vi "popUPSeleccionReceta.vi"(9 "ingresarLote":string="numLote", 10 "ingresarSteelGrade":string="numSteelGrade", 11 "ingresarOD":string="numeroOD") -> (1 "idReceta":string, 2 "recetaSeleccionadaDeLaLista":string, 3 "Listo SeleccionListaDeReceta":bool=TRUE)   [LabVIEW 2014]
panel:
  in  "listaRecetas":i32(listbox)
  in  "textoFinCarga":string="Gracias por ingresar los datos del producto"
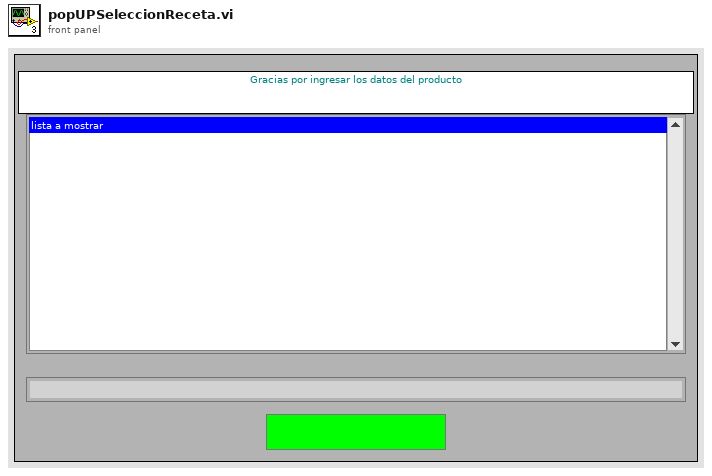
[diagram p1: front panel]
types:
  T1 = enum8{"Enabled", "Disabled", "Disabled and Grayed Out"}
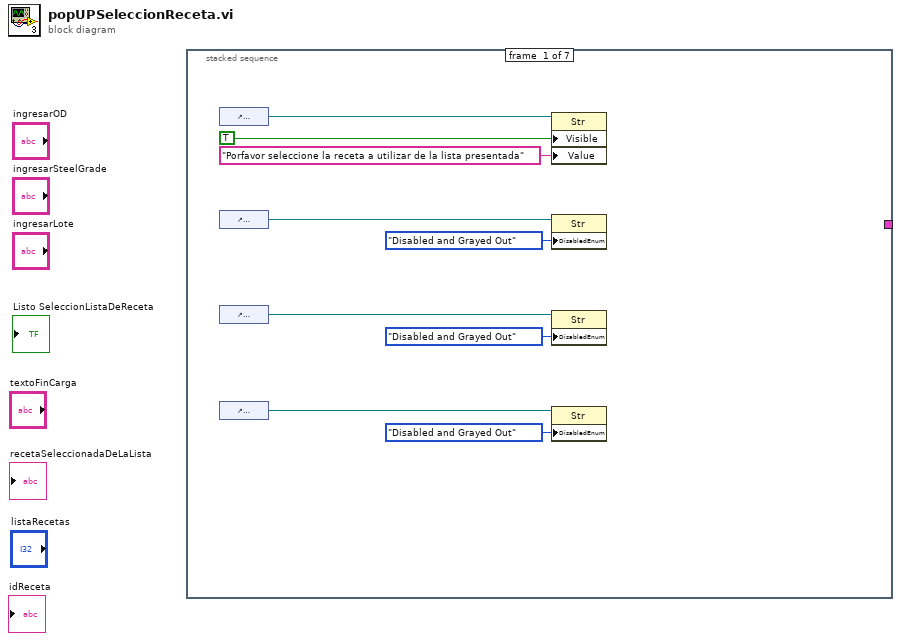
[diagram p0: block diagram]
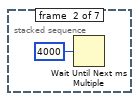
[diagram p2: hidden frame]
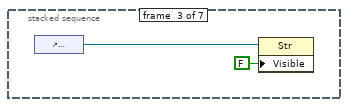
[diagram p3: hidden frame]
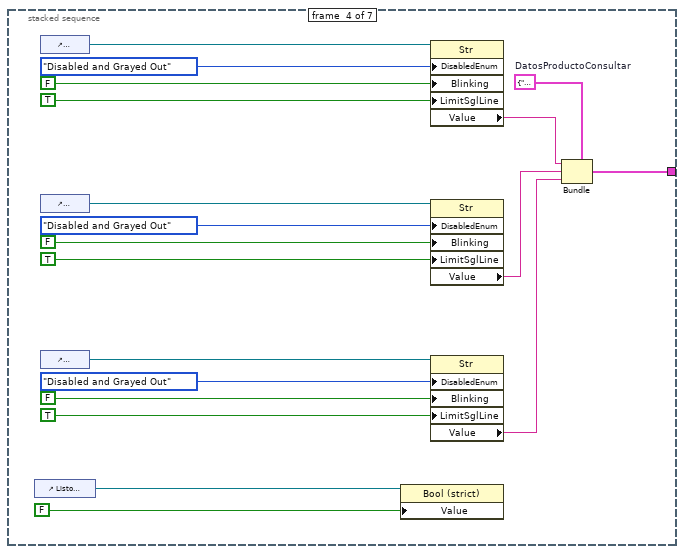
[diagram p4: hidden frame]
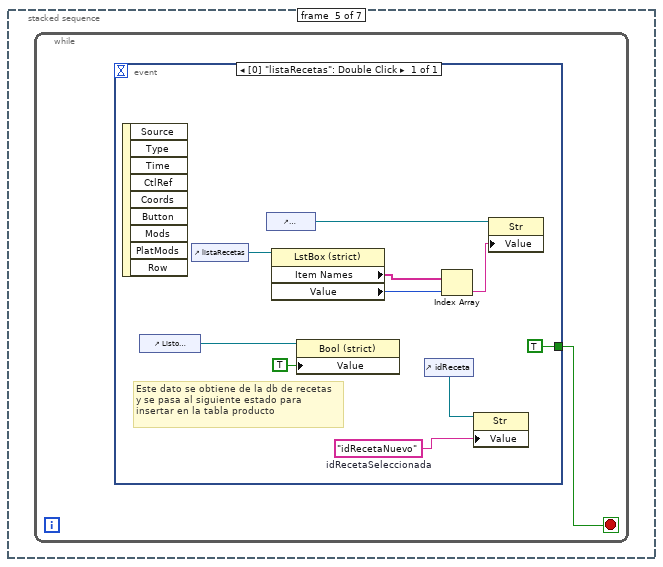
[diagram p5: hidden frame]
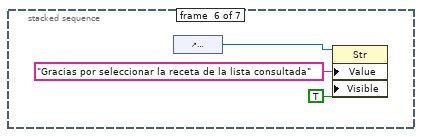
[diagram p6: hidden frame]
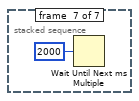
[diagram p7: hidden frame]
diagram:
  n1 = stacked-sequence {
    tunnel: [_ _ _ w13 _ _ _] -> _
    frame #0 {
      n2 = control-ref of="textoFinCarga"() -> (w9:refnum<vi>)
      n3 = control-ref of="ingresarOD"() -> (w6:refnum<vi>)
      n4 = control-ref of="ingresarSteelGrade"() -> (w5:refnum<vi>)
      n5 = control-ref of="ingresarLote"() -> (w4:refnum<vi>)
      n6 = property class="Str"(reference=w9, "Visible"=TRUE, "Value"="Porfavor seleccione la receta a utilizar de la lista presentada") -> ()  [unwired: 1 in, 2 out]
      n7 = property class="Str"(reference=w6, "DisabledEnum"=T1."Disabled and Grayed Out" ("Disabled")) -> ()  [unwired: 1 in, 2 out]
      n8 = property class="Str"(reference=w5, "DisabledEnum"=T1."Disabled and Grayed Out" ("Disabled")) -> ()  [unwired: 1 in, 2 out]
      n9 = property class="Str"(reference=w4, "DisabledEnum"=T1."Disabled and Grayed Out" ("Disabled")) -> ()  [unwired: 1 in, 2 out]
    }
    frame #1 {
      n10 = Wait Until Next ms Multiple(millisecond multiple=u32 4000) -> ()  [unwired: 1 out]
    }
    frame #2 {
      n11 = control-ref of="textoFinCarga"() -> (w12:refnum<vi>)
      n12 = property class="Str"(reference=w12, "Visible"=FALSE) -> ()  [unwired: 1 in, 2 out]
    }
    frame #3 {
      w14 = cluster{"OD":string, "SG":string, "LT":string} {"OD"="", "SG"="", "LT"=""}  # DatosProductoConsultar
      n13 = control-ref of="Listo SeleccionListaDeReceta"() -> (w19:refnum<vi>)
      n14 = control-ref of="ingresarOD"() -> (w31:refnum<vi>)
      n15 = control-ref of="ingresarSteelGrade"() -> (w29:refnum<vi>)
      n16 = control-ref of="ingresarLote"() -> (w27:refnum<vi>)
      n17 = property class="Bool (strict)"(reference=w19, "Value"=FALSE) -> ()  [unwired: 1 in, 2 out]
      n18 = property class="Str"(reference=w31, "DisabledEnum"=T1."Disabled and Grayed Out" ("Disabled"), "Blinking"=FALSE, "LimitSglLine"=TRUE ("Limit To Single Line?")) -> ("Value"=w17:string)  [unwired: 1 in, 2 out]
      n19 = property class="Str"(reference=w29, "DisabledEnum"=T1."Disabled and Grayed Out" ("Disabled"), "Blinking"=FALSE, "LimitSglLine"=TRUE ("Limit To Single Line?")) -> ("Value"=w16:string)  [unwired: 1 in, 2 out]
      n20 = property class="Str"(reference=w27, "DisabledEnum"=T1."Disabled and Grayed Out" ("Disabled"), "Blinking"=FALSE, "LimitSglLine"=TRUE ("Limit To Single Line?")) -> ("Value"=w15:string)  [unwired: 1 in, 2 out]
      n21 = Bundle(cluster=w14, "OD"=w17, "SG"=w16, "LT"=w15) -> (w13:cluster{"OD":string, "SG":string, "LT":string})
    }
    frame #4 {
      n22 = while {
        stop <- w32 stop-if-true
        n23 = event shown="[0] \"listaRecetas\": Double Click" {
          selector: _ -> [_]
          dyn-events: _ -> [_]
          timeout: _ -> [_]
          tunnel: [TRUE] -> w32
          event "listaRecetas": Double Click {
            w33 = "idRecetaNuevo"  # idRecetaSeleccionada
            # "Este dato se obtiene de la db de recetas\ny se pasa al siguiente estado para\ninsertar en la tabla producto"
            n24 = event-data() -> ()  [unwired: 1 in, 9 out]
            n25 = control-ref of="Listo SeleccionListaDeReceta"() -> (w41:refnum<vi>)
            n26 = control-ref of="listaRecetas"() -> (w39:refnum<vi>)
            n27 = control-ref of="recetaSeleccionadaDeLaLista"() -> (w35:refnum<vi>)
            n28 = property class="LstBox (strict)"(reference=w39) -> ("Item Names"=w38:string[], "Value"=w37:i32)  [unwired: 1 in, 2 out]
            n29 = property class="Bool (strict)"(reference=w41, "Value"=TRUE) -> ()  [unwired: 1 in, 2 out]
            n30 = control-ref of="idReceta"() -> (w34:refnum<vi>)
            n31 = Index Array(array=w38, index=w37) -> (element=w36:string)
            n32 = property class="Str"(reference=w34, "Value"=w33) -> ()  [unwired: 1 in, 2 out]
            n33 = property class="Str"(reference=w35, "Value"=w36) -> ()  [unwired: 1 in, 2 out]
          }
        }
      }
    }
    frame #5 {
      n34 = control-ref of="textoFinCarga"() -> (w45:refnum<vi>)
      n35 = property class="Str"(reference=w45, "Value"="Gracias por seleccionar la receta de la lista consultada", "Visible"=TRUE) -> ()  [unwired: 1 in, 2 out]
    }
    frame #6 {
      n36 = Wait Until Next ms Multiple(millisecond multiple=u32 2000) -> ()  [unwired: 1 out]
    }
  }
